vi "Untitled 1.vi"() -> ()   [LabVIEW 2016]
panel:
  in  "Trigg":bool
  in  "Setup":bool
  in  "Values start":u16(ring)=5 items=["External rising edge"=1, "Single shot internal rising edge"=3, "Single shot"=5]
  in  "Delay H (0 s)":dbl format="%#_16g"
  in  "Delay G (0 s)":dbl format="%#_16g"
  in  "Delay F (0 s)":dbl format="%#_16g"
  in  "Delay E (0 s)":dbl format="%#_16g"
  in  "Delay D (0 s)":dbl format="%#_16g"
  in  "Delay C (0 s)":dbl format="%#_16g"
  in  "H":bool
  in  "G":bool
  in  "F":bool
  in  "E":bool
  in  "D":bool
  in  "C":bool
  in  "Delay B (0 s)":dbl format="%#_16g"
  in  "B":bool
  in  "stop":bool
  in  "Delay A (0 s)":dbl format="%#_16g"
  out "VISA resource name out":refnum<visa-resource-name>
  in  "A":bool
  out "error out":errorcluster
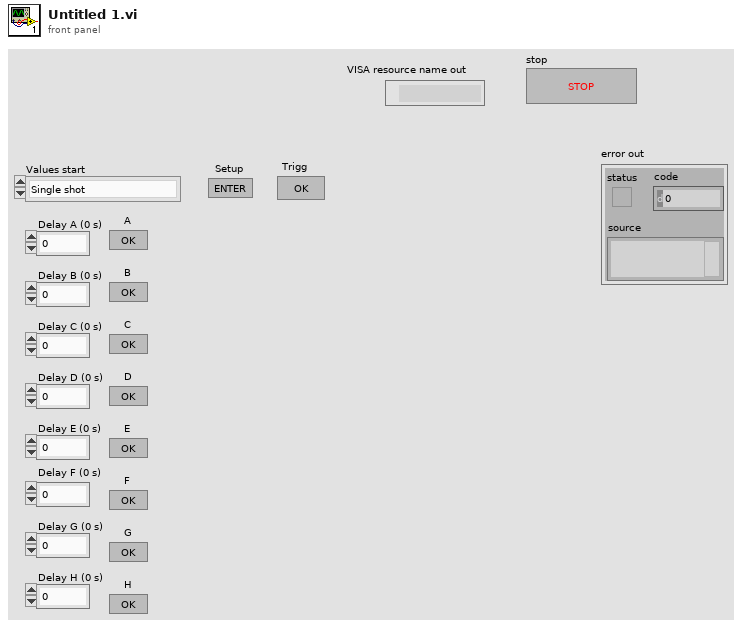
[diagram p1: front panel]
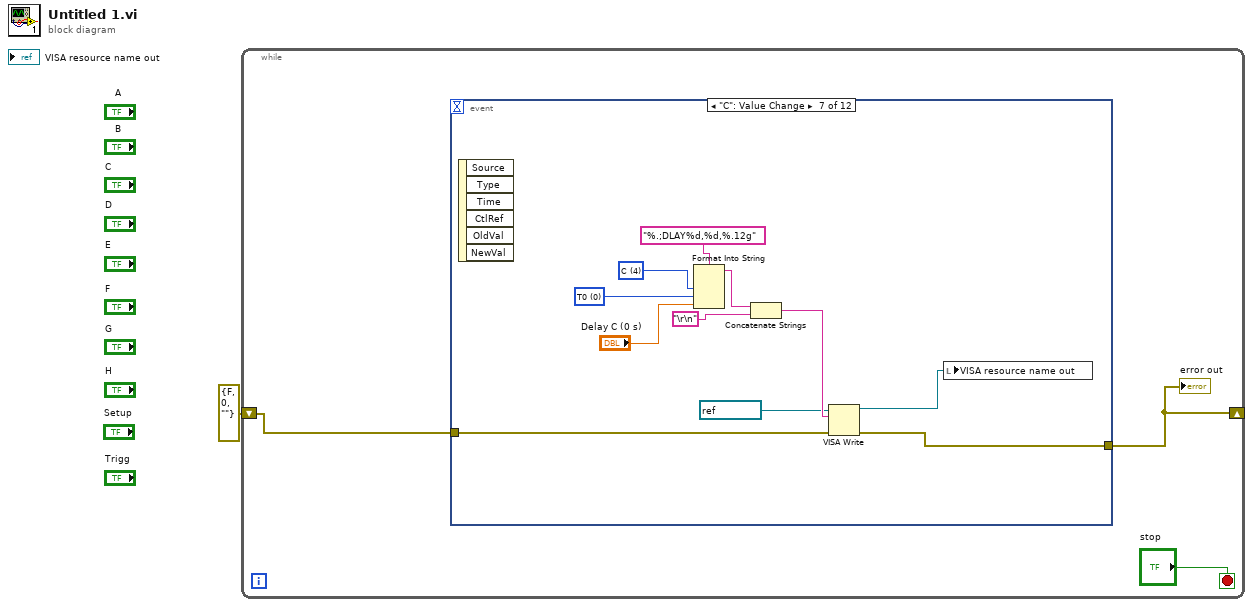
[diagram p0: block diagram]
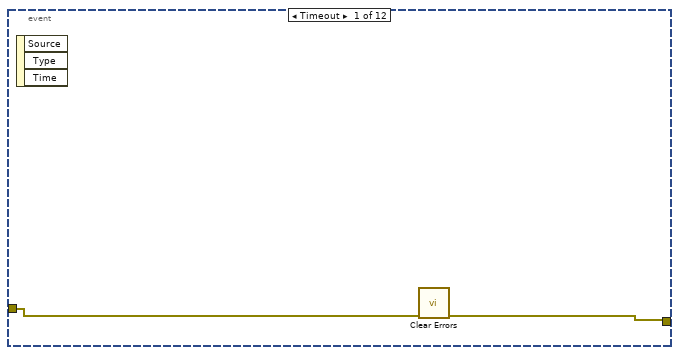
[diagram p2: hidden frame]
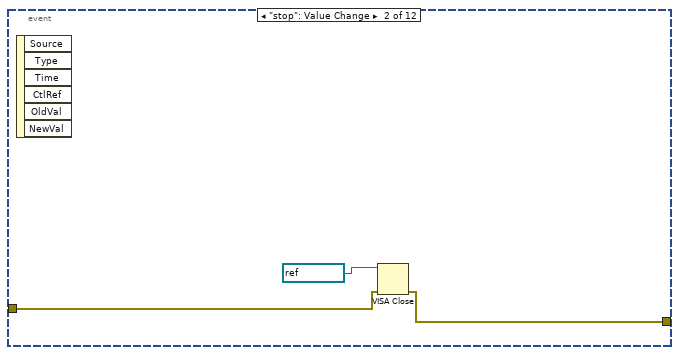
[diagram p3: hidden frame]
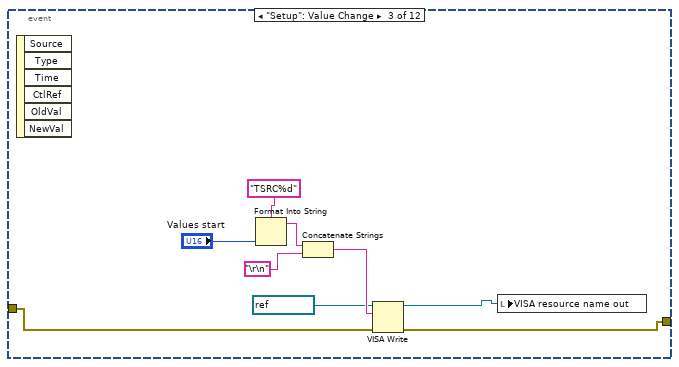
[diagram p4: hidden frame]
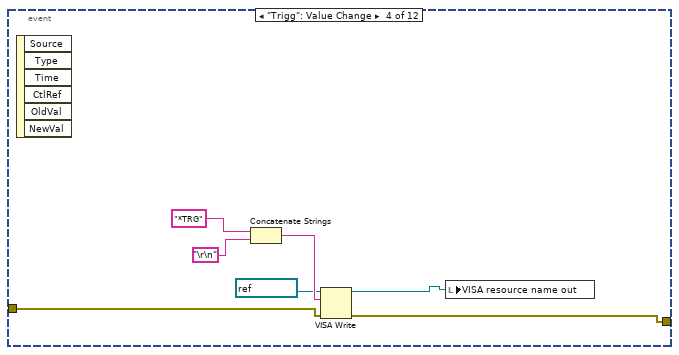
[diagram p5: hidden frame]
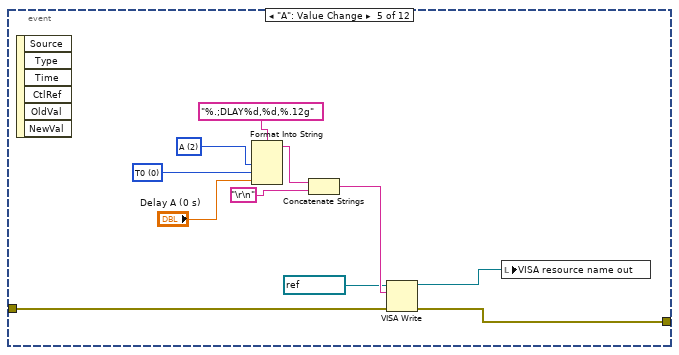
[diagram p6: hidden frame]
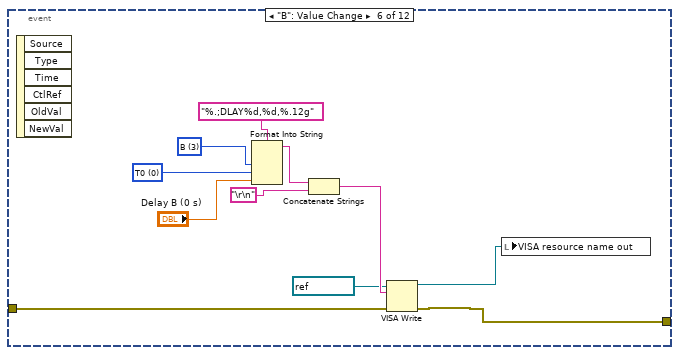
[diagram p7: hidden frame]
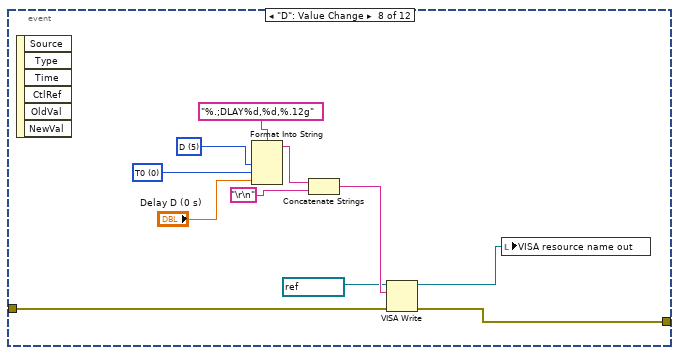
[diagram p8: hidden frame]
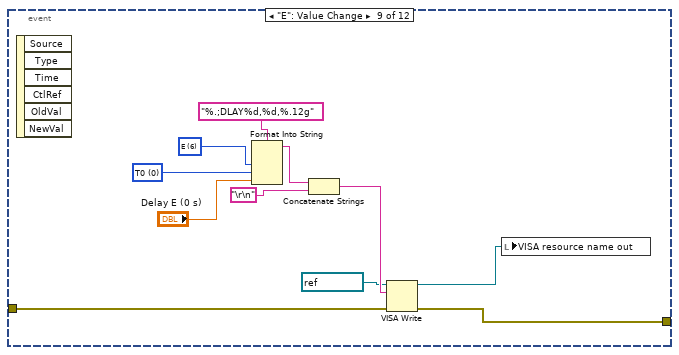
[diagram p9: hidden frame]
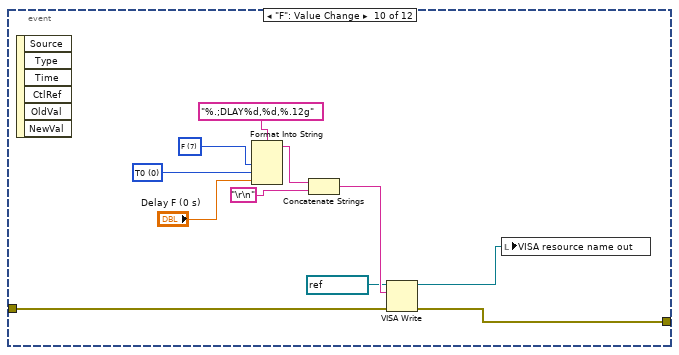
[diagram p10: hidden frame]
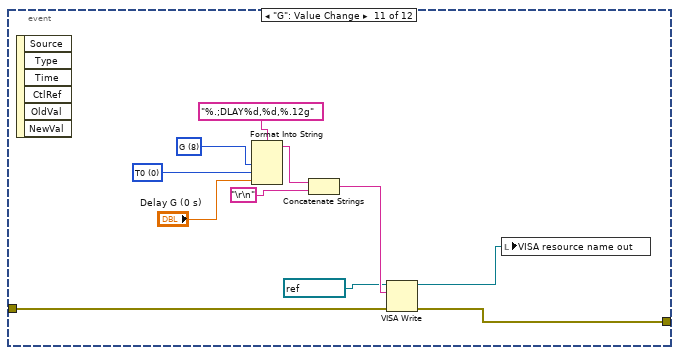
[diagram p11: hidden frame]
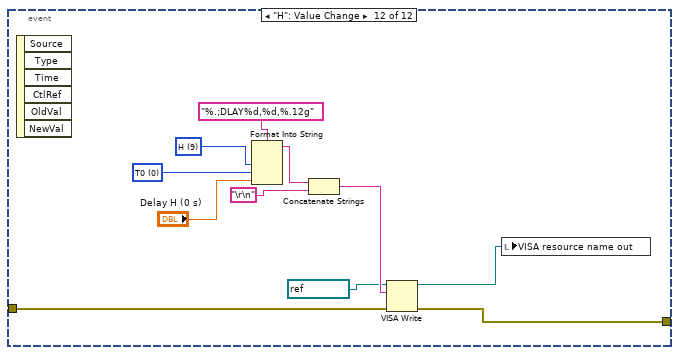
[diagram p12: hidden frame]
diagram:
  n1 = while {
    shift-right: [w4] -> _
    shift-left: errorcluster {"status"=FALSE, "code"=0, "source"=""} ("error out") -> [w2]
    stop <- "stop" stop-if-true
    n2 = event shown="[6] \"C\": Value Change" {
      selector: _ -> [_ _ _ _ _ _ _ _ _ _ _ _]
      dyn-events: _ -> [_ _ _ _ _ _ _ _ _ _ _ _]
      timeout: _ -> [_ _ _ _ _ _ _ _ _ _ _ _]
      tunnel: [w5 w8 w13 w23 w28 w39 w50 w61 w72 w83 w94 w105] -> w4
      tunnel: w2 -> [w6 w9 w11 w21 w29 w40 w51 w62 w73 w84 w95 w106]
      event Timeout {
        n3 = event-data() -> ()  [unwired: 1 in, 3 out]
        n4 = call <vilib>:"Clear Errors.vi"("error in (no error)"=w6) -> ("error out"=w5:errorcluster)  [unwired: 5 in, 1 out]
      }
      event "stop": Value Change {
        n5 = event-data() -> ()  [unwired: 1 in, 6 out]
        n6 = VISA Close(VISA resource name=refnum<visa-resource-name> "DG645", error in (no error)=w9) -> (error out=w8:errorcluster)
      }
      event "Setup": Value Change {
        n7 = event-data() -> ()  [unwired: 1 in, 6 out]
        n8 = Format Into String(format string="TSRC%d", "Values start") -> (resulting string=w16:string)  [unwired: 2 in, 1 out]
        n9 = Concatenate Strings(w16, "\r\n") -> (w18:string)
        n10 = VISA Write(VISA resource name=refnum<visa-resource-name> "DG645", write buffer=w18, error in (no error)=w11) -> (VISA resource name out=w12:refnum<visa-resource-name>, error out=w13:errorcluster)  [unwired: 1 out]
        n11 = local write "VISA resource name out"(w12) -> ()
      }
      event "Trigg": Value Change {
        n12 = event-data() -> ()  [unwired: 1 in, 6 out]
        n13 = Concatenate Strings("*TRG" ("string"), "\r\n") -> (w22:string)
        n14 = VISA Write(VISA resource name=refnum<visa-resource-name> "DG645", write buffer=w22, error in (no error)=w21) -> (VISA resource name out=w25:refnum<visa-resource-name>, error out=w23:errorcluster)  [unwired: 1 out]
        n15 = local write "VISA resource name out"(w25) -> ()
      }
      event "A": Value Change {
        w30 = u16 0 items=["T0"=0, "A"=2, "B"=3, "C"=4, "D"=5, "E"=6, "F"=7, "G"=8, "H"=9] ("Reference Channel (0:T0)")
        w35 = u16 2 items=["A"=2, "B"=3, "C"=4, "D"=5, "E"=6, "F"=7, "G"=8, "H"=9] ("Channel to Modify (2:A)")
        n16 = event-data() -> ()  [unwired: 1 in, 6 out]
        n17 = Format Into String(format string="%.;DLAY%d,%d,%.12g" ("Set Delay Command"), w35, w30, "Delay A (0 s)") -> (resulting string=w33:string)  [unwired: 2 in, 1 out]
        n18 = Concatenate Strings(w33, "\r\n") -> (w32:string)
        n19 = VISA Write(VISA resource name=refnum<visa-resource-name> "DG645", write buffer=w32, error in (no error)=w29) -> (VISA resource name out=w27:refnum<visa-resource-name>, error out=w28:errorcluster)  [unwired: 1 out]
        n20 = local write "VISA resource name out"(w27) -> ()
      }
      event "B": Value Change {
        w41 = u16 0 items=["T0"=0, "A"=2, "B"=3, "C"=4, "D"=5, "E"=6, "F"=7, "G"=8, "H"=9] ("Reference Channel (0:T0)")
        w46 = u16 3 items=["A"=2, "B"=3, "C"=4, "D"=5, "E"=6, "F"=7, "G"=8, "H"=9] ("Channel to Modify (2:A)")
        n21 = event-data() -> ()  [unwired: 1 in, 6 out]
        n22 = Format Into String(format string="%.;DLAY%d,%d,%.12g" ("Set Delay Command"), w46, w41, "Delay B (0 s)") -> (resulting string=w44:string)  [unwired: 2 in, 1 out]
        n23 = Concatenate Strings(w44, "\r\n") -> (w43:string)
        n24 = VISA Write(VISA resource name=refnum<visa-resource-name> "DG645", write buffer=w43, error in (no error)=w40) -> (VISA resource name out=w38:refnum<visa-resource-name>, error out=w39:errorcluster)  [unwired: 1 out]
        n25 = local write "VISA resource name out"(w38) -> ()
      }
      event "C": Value Change {
        w52 = u16 0 items=["T0"=0, "A"=2, "B"=3, "C"=4, "D"=5, "E"=6, "F"=7, "G"=8, "H"=9] ("Reference Channel (0:T0)")
        w57 = u16 4 items=["A"=2, "B"=3, "C"=4, "D"=5, "E"=6, "F"=7, "G"=8, "H"=9] ("Channel to Modify (2:A)")
        n26 = event-data() -> ()  [unwired: 1 in, 6 out]
        n27 = Format Into String(format string="%.;DLAY%d,%d,%.12g" ("Set Delay Command"), w57, w52, "Delay C (0 s)") -> (resulting string=w55:string)  [unwired: 2 in, 1 out]
        n28 = Concatenate Strings(w55, "\r\n") -> (w54:string)
        n29 = VISA Write(VISA resource name=refnum<visa-resource-name> "DG645", write buffer=w54, error in (no error)=w51) -> (VISA resource name out=w49:refnum<visa-resource-name>, error out=w50:errorcluster)  [unwired: 1 out]
        n30 = local write "VISA resource name out"(w49) -> ()
      }
      event "D": Value Change {
        w63 = u16 0 items=["T0"=0, "A"=2, "B"=3, "C"=4, "D"=5, "E"=6, "F"=7, "G"=8, "H"=9] ("Reference Channel (0:T0)")
        w68 = u16 5 items=["A"=2, "B"=3, "C"=4, "D"=5, "E"=6, "F"=7, "G"=8, "H"=9] ("Channel to Modify (2:A)")
        n31 = event-data() -> ()  [unwired: 1 in, 6 out]
        n32 = Format Into String(format string="%.;DLAY%d,%d,%.12g" ("Set Delay Command"), w68, w63, "Delay D (0 s)") -> (resulting string=w66:string)  [unwired: 2 in, 1 out]
        n33 = Concatenate Strings(w66, "\r\n") -> (w65:string)
        n34 = VISA Write(VISA resource name=refnum<visa-resource-name> "DG645", write buffer=w65, error in (no error)=w62) -> (VISA resource name out=w60:refnum<visa-resource-name>, error out=w61:errorcluster)  [unwired: 1 out]
        n35 = local write "VISA resource name out"(w60) -> ()
      }
      event "E": Value Change {
        w74 = u16 0 items=["T0"=0, "A"=2, "B"=3, "C"=4, "D"=5, "E"=6, "F"=7, "G"=8, "H"=9] ("Reference Channel (0:T0)")
        w79 = u16 6 items=["A"=2, "B"=3, "C"=4, "D"=5, "E"=6, "F"=7, "G"=8, "H"=9] ("Channel to Modify (2:A)")
        n36 = event-data() -> ()  [unwired: 1 in, 6 out]
        n37 = Format Into String(format string="%.;DLAY%d,%d,%.12g" ("Set Delay Command"), w79, w74, "Delay E (0 s)") -> (resulting string=w77:string)  [unwired: 2 in, 1 out]
        n38 = Concatenate Strings(w77, "\r\n") -> (w76:string)
        n39 = VISA Write(VISA resource name=refnum<visa-resource-name> "DG645", write buffer=w76, error in (no error)=w73) -> (VISA resource name out=w71:refnum<visa-resource-name>, error out=w72:errorcluster)  [unwired: 1 out]
        n40 = local write "VISA resource name out"(w71) -> ()
      }
      event "F": Value Change {
        w85 = u16 0 items=["T0"=0, "A"=2, "B"=3, "C"=4, "D"=5, "E"=6, "F"=7, "G"=8, "H"=9] ("Reference Channel (0:T0)")
        w90 = u16 7 items=["A"=2, "B"=3, "C"=4, "D"=5, "E"=6, "F"=7, "G"=8, "H"=9] ("Channel to Modify (2:A)")
        n41 = event-data() -> ()  [unwired: 1 in, 6 out]
        n42 = Format Into String(format string="%.;DLAY%d,%d,%.12g" ("Set Delay Command"), w90, w85, "Delay F (0 s)") -> (resulting string=w88:string)  [unwired: 2 in, 1 out]
        n43 = Concatenate Strings(w88, "\r\n") -> (w87:string)
        n44 = VISA Write(VISA resource name=refnum<visa-resource-name> "DG645", write buffer=w87, error in (no error)=w84) -> (VISA resource name out=w82:refnum<visa-resource-name>, error out=w83:errorcluster)  [unwired: 1 out]
        n45 = local write "VISA resource name out"(w82) -> ()
      }
      event "G": Value Change {
        w96 = u16 0 items=["T0"=0, "A"=2, "B"=3, "C"=4, "D"=5, "E"=6, "F"=7, "G"=8, "H"=9] ("Reference Channel (0:T0)")
        w101 = u16 8 items=["A"=2, "B"=3, "C"=4, "D"=5, "E"=6, "F"=7, "G"=8, "H"=9] ("Channel to Modify (2:A)")
        n46 = event-data() -> ()  [unwired: 1 in, 6 out]
        n47 = Format Into String(format string="%.;DLAY%d,%d,%.12g" ("Set Delay Command"), w101, w96, "Delay G (0 s)") -> (resulting string=w99:string)  [unwired: 2 in, 1 out]
        n48 = Concatenate Strings(w99, "\r\n") -> (w98:string)
        n49 = VISA Write(VISA resource name=refnum<visa-resource-name> "DG645", write buffer=w98, error in (no error)=w95) -> (VISA resource name out=w93:refnum<visa-resource-name>, error out=w94:errorcluster)  [unwired: 1 out]
        n50 = local write "VISA resource name out"(w93) -> ()
      }
      event "H": Value Change {
        w107 = u16 0 items=["T0"=0, "A"=2, "B"=3, "C"=4, "D"=5, "E"=6, "F"=7, "G"=8, "H"=9] ("Reference Channel (0:T0)")
        w112 = u16 9 items=["A"=2, "B"=3, "C"=4, "D"=5, "E"=6, "F"=7, "G"=8, "H"=9] ("Channel to Modify (2:A)")
        n51 = event-data() -> ()  [unwired: 1 in, 6 out]
        n52 = Format Into String(format string="%.;DLAY%d,%d,%.12g" ("Set Delay Command"), w112, w107, "Delay H (0 s)") -> (resulting string=w110:string)  [unwired: 2 in, 1 out]
        n53 = Concatenate Strings(w110, "\r\n") -> (w109:string)
        n54 = VISA Write(VISA resource name=refnum<visa-resource-name> "DG645", write buffer=w109, error in (no error)=w106) -> (VISA resource name out=w104:refnum<visa-resource-name>, error out=w105:errorcluster)  [unwired: 1 out]
        n55 = local write "VISA resource name out"(w104) -> ()
      }
    }
    "error out" <- w4
  }
